vi "OPM.ThorlabsPM400.SetResource.vi"(8 "error in (no error)":errorcluster, 10 "Resource":T1, 11 "OPM.ThorlabsPM400 in":refnum<class "OPM.ThorlabsPM400.lvclass">) -> (0 "error out":errorcluster, 3 "OPM.ThorlabsPM400 out":refnum<class "OPM.ThorlabsPM400.lvclass">)   [LabVIEW 2017, in "OPM.ThorlabsPM400.lvclass"]
uses:
  OPM.ThorlabsPM400.lvclass
  Typedefs/Resource--Cluster.ctl
  OPM.ThorlabsPM400.lvclass/OPM.ThorlabsPM400.ctl
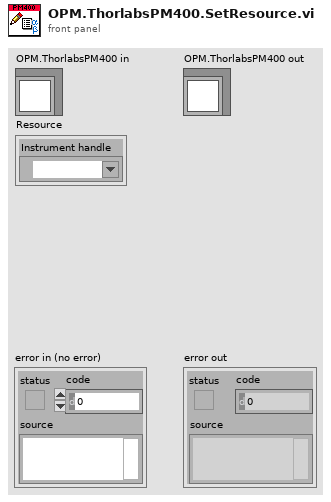
[diagram p1: front panel]
types:
  T1 = typedef "OPM.ThorlabsPM400.lvclass/Resource--Cluster.ctl" = cluster{"Instrument handle":refnum<visa-resource-name>}
  T2 = typedef "OPM.ThorlabsPM400.lvclass/PrivateData--Ref.ctl" = refnum<data-value>
  T3 = typedef "OPM.ThorlabsPM400.lvclass/PrivateData--Cluster.ctl" = cluster{"Resource":T1}
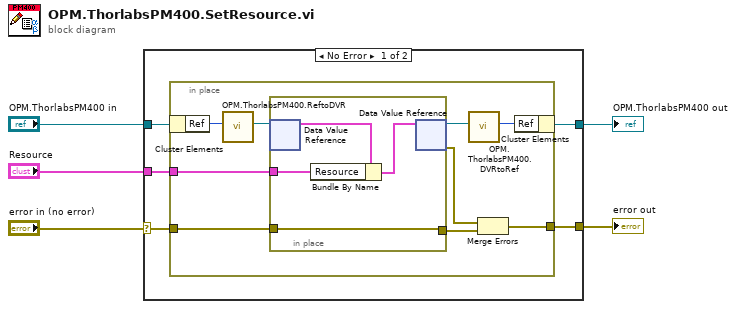
[diagram p0: block diagram]
diagram:
  n1 = case shown="No Error" "error in (no error)" {
    selector: "error in (no error)" -> [w7 w25]
    tunnel: [w6 w25] -> w4
    tunnel: [w9 w24] -> w2
    tunnel: "OPM.ThorlabsPM400 in" -> [w10 w24]
    tunnel: "Resource" -> [w8 _]
    frame No Error {
      n2 = in-place {
        in-place-border: w8 -> [w16]
        in-place-border: w7 -> [w13]
        in-place-border: [w11] -> w6
        n3 = in-place-cluster #1(w10) -> ("Ref"=w19:u32)
        n4 = call "OPM.ThorlabsPM400.ReftoDVR.vi"("Ref"=w19) -> ("Ref"=w17:T2)  [unwired: 10 in]
        n5 = in-place {
          in-place-border: w16 -> [w21]
          in-place-border: [w20] -> w12
          in-place-border: w13 -> [w20]
          n6 = in-place-dvr #2(w17) -> (w23:T3)  [unwired: 1 out]
          n7 = Bundle By Name(cluster=w23, "Resource"=w21) -> (w22:T3)
          n8 = in-place-dvr #2(w22) -> (w15:T2, w14:errorcluster)
        }
        n9 = call "OPM.ThorlabsPM400.DVRtoRef.vi"("Ref"=w15) -> ("Ref"=w18:u32)  [unwired: 10 in]
        n10 = Merge Errors(w14, w12) -> (w11:errorcluster)
        n11 = in-place-cluster #1("Ref"=w18) -> (w9:refnum<class "OPM.ThorlabsPM400.lvclass">)
      }
    }
    frame Error {
    }
  }
  "error out" <- w4
  "OPM.ThorlabsPM400 out" <- w2
